vi "Video record flag clear.vi"   [LabVIEW 2013]
uses:
  typedefs/Functions enum.ctl
types:
  T1 = typedef "Functions enum.ctl" = enum16{"Create", "Start", "Write", "Stop", "Clear"}
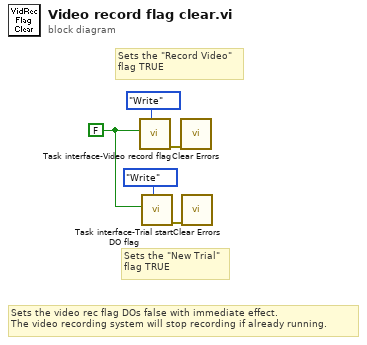
[diagram p0: block diagram]
diagram:
  w1 = FALSE ("DO value")
  # "Sets the video rec flag DOs false with immediate effect.\nThe video recording system will stop recording if already running."
  # "Sets the \"New Trial\"\nflag TRUE"
  # "Sets the \"Record Video\"\nflag TRUE"
  n1 = call "Task interface-Video record flag.vi"("Function"=Functions_enum."Write", "DO value"=w1) -> ("error out"=w3:errorcluster)  [unwired: 9 in]
  n2 = call "Task interface-Trial start DO flag.vi"("Function"=Functions_enum."Write", "DO value"=w1) -> ("error out"=w5:errorcluster)  [unwired: 9 in]
  n3 = call <vilib>:"Clear Errors.vi"("error in (no error)"=w3) -> ()  [unwired: 6 in, 1 out]
  n4 = call <vilib>:"Clear Errors.vi"("error in (no error)"=w5) -> ()  [unwired: 6 in, 1 out]
